vi "SMC_SetDim.vi"(8 "error in (no error)":errorcluster, 11 "Dimension":u8) -> (0 "error out":errorcluster)   [LabVIEW 2015]
uses:
  SMC_SubVIs.llb/SMC_ManagerMode.ctl
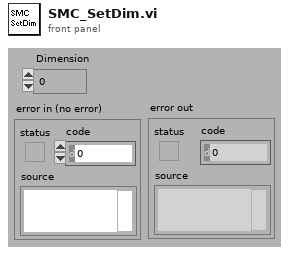
[diagram p1: front panel]
types:
  T1 = typedef "SMC_ManagerMode.ctl" = enum16{"Init", "Get", "SetPosition", "SetStatus", "SetMoving", "SetControllerNr"}
  T2 = typedef "SMC Paras.ctl" = cluster{"VENUS Language":T3, "Number of Axis":u8, "Controller Nr":u8, "Simulation":bool}
  T3 = typedef "VENUSNr.ctl" = enum16{"VENUS 2", "VENUS 1"}
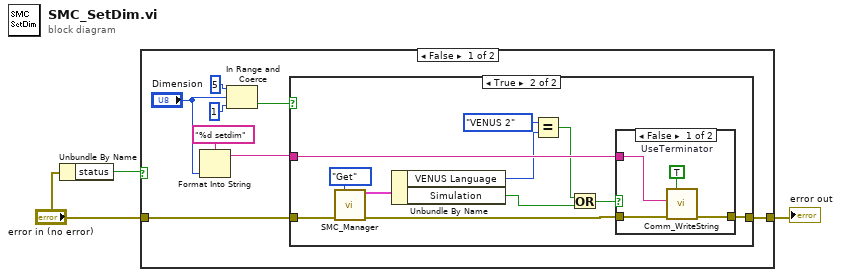
[diagram p0: block diagram]
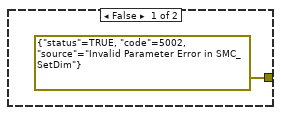
[diagram p2: hidden frame]
diagram:
  n1 = Unbundle By Name("error in (no error)") -> ("status"=w3:bool)
  n2 = case shown="False" w3 {
    tunnel: "error in (no error)" -> [w11 w29]
    tunnel: [w10 w29] -> w1
    frame False {
      n3 = Format Into String(format string="%d setdim" ("Format String"), "Dimension") -> (resulting string=w4:string)  [unwired: 2 in, 1 out]
      n4 = In Range and Coerce(upper limit=u8 5 ("hi"), x="Dimension", lower limit=u8 1 ("lo")) -> (In Range?=w7:bool)  [unwired: 1 out]
      n5 = case shown="True" w7 {
        tunnel: w11 -> [_ w22]
        tunnel: [errorcluster {"status"=TRUE, "code"=5002, "source"="Invalid Parameter Error in SMC_SetDim"} ("t") w19] -> w10
        tunnel: w4 -> [_ w21]
        frame False {
        }
        frame True {
          n6 = call "SMC_Manager.vi"("Mode"=SMC_ManagerMode."Get", "error in (no error)"=w22) -> ("SMC Parameter Out"=w15:T2, "error out"=w20:errorcluster)  [unwired: 9 in, 3 out]
          n7 = Unbundle By Name(w15) -> ("VENUS Language"=w14:T3, "Simulation"=w13:bool)
          n8 = Equal?(x=enum16{"VENUS 2", "VENUS 1"}."VENUS 2", y=w14) -> (x = y?=w16:bool)
          n9 = Or(x=w16, y=w13) -> (x .or. y?=w18:bool)
          n10 = case shown="False" w18 {
            tunnel: w21 -> [w27 _]
            tunnel: w20 -> [w26 w28]
            tunnel: [w25 w28] -> w19
            frame False {
              w24 = TRUE  # UseTerminator
              n11 = call "Comm_WriteString.vi"("string to write"=w27, "error in (no error)"=w26, "UseTerminator"=w24) -> ("error out"=w25:errorcluster)  [unwired: 8 in]
            }
            frame True {
            }
          }
        }
      }
    }
    frame True {
      # "Error, do nothing"
    }
  }
  "error out" <- w1
